vi "Util Hex String to Ascii String.vi"(8 "error in (no error)":errorcluster, 11 "Hex String":string) -> (0 "error out":errorcluster, 3 "Ascii String":string)   [LabVIEW 2017, in "xHelper.lvlib"]
uses:
  xHelper.lvlib
panel:
  out "U8 Array":u8[](array[numeric]) format="%x"
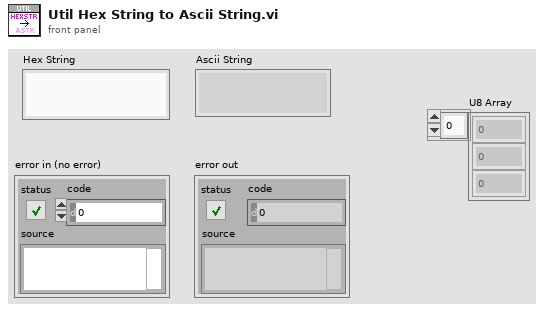
[diagram p1: front panel]
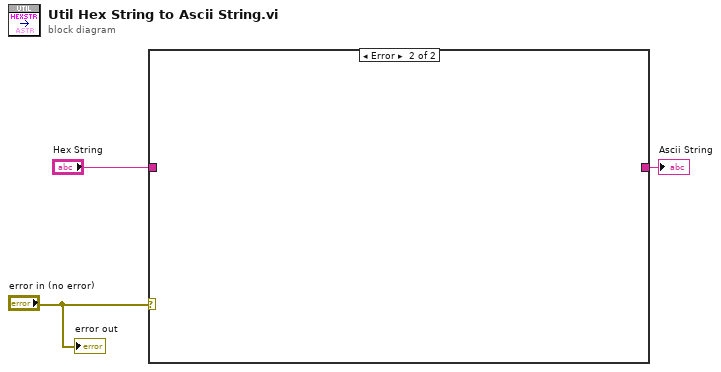
[diagram p0: block diagram]
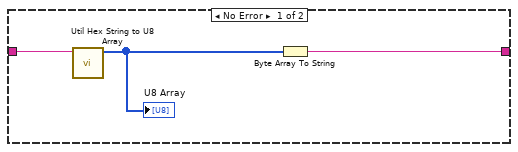
[diagram p2: hidden frame]
diagram:
  n1 = case shown="Error" "error in (no error)" {
    tunnel: "Hex String" -> [w6 _]
    tunnel: [w4 _] -> w1
    frame No Error {
      n2 = call "Util Hex String to U8 Array.vi"("Hex String"=w6) -> ("U8 Array"=w5:u8[])  [unwired: 9 in, 1 out]
      "U8 Array" <- w5
      n3 = Byte Array To String(unsigned byte array=w5) -> (string=w4:string)
    }
    frame Error {
    }
  }
  "Ascii String" <- w1
  "error out" <- "error in (no error)"
